vi "Create Bar.vi"(6 "Draw Mode":T1(ring)=enum."Quads", 7 "3D Bar Property":T2, 8 "error in (no error)":errorcluster, 10 "Plot Representation In":T4, 11 "Plot Object In":refnum<vi>) -> (0 "error out":errorcluster, 2 "Plot Representation Out":T4, 3 "Plot Object Out":refnum<vi>, 4 "Sector Object Out":refnum<vi>, 5 "Bar Drawable":refnum<vi>)   [LabVIEW 2017, in "3D Bar.lvclass"]
uses:
  <vilib>/Math Plots/3D Math Plots/3D Bar/3D Bar/3D Bar.lvclass
  <vilib>/Math Plots/3D Math Plots/3D Plot/3D Plot/Typedef/Plot Representation.ctl
  <vilib>/Math Plots/3D Math Plots/3D Plot/3D Plot/Typedef/Range Clusters.ctl
  <vilib>/Math Plots/3D Math Plots/3D Plot/3D Plot/Typedef/Mesh Data.ctl
  <vilib>/Math Plots/3D Math Plots/3D Bar/3D Bar/Typedef/3D Bar Property.ctl
  <vilib>/Math Plots/3D Math Plots/3D Plot/3D Plot/Typedef/Line Type.ctl
  <vilib>/picture/3D Picture Control/Object/Create Object (name).vi
  <vilib>/picture/3D Picture Control/NI_3D Picture Control.lvlib
  <vilib>/Math Plots/3D Math Plots/3D Plot/3D Plot/3D Plot.lvclass
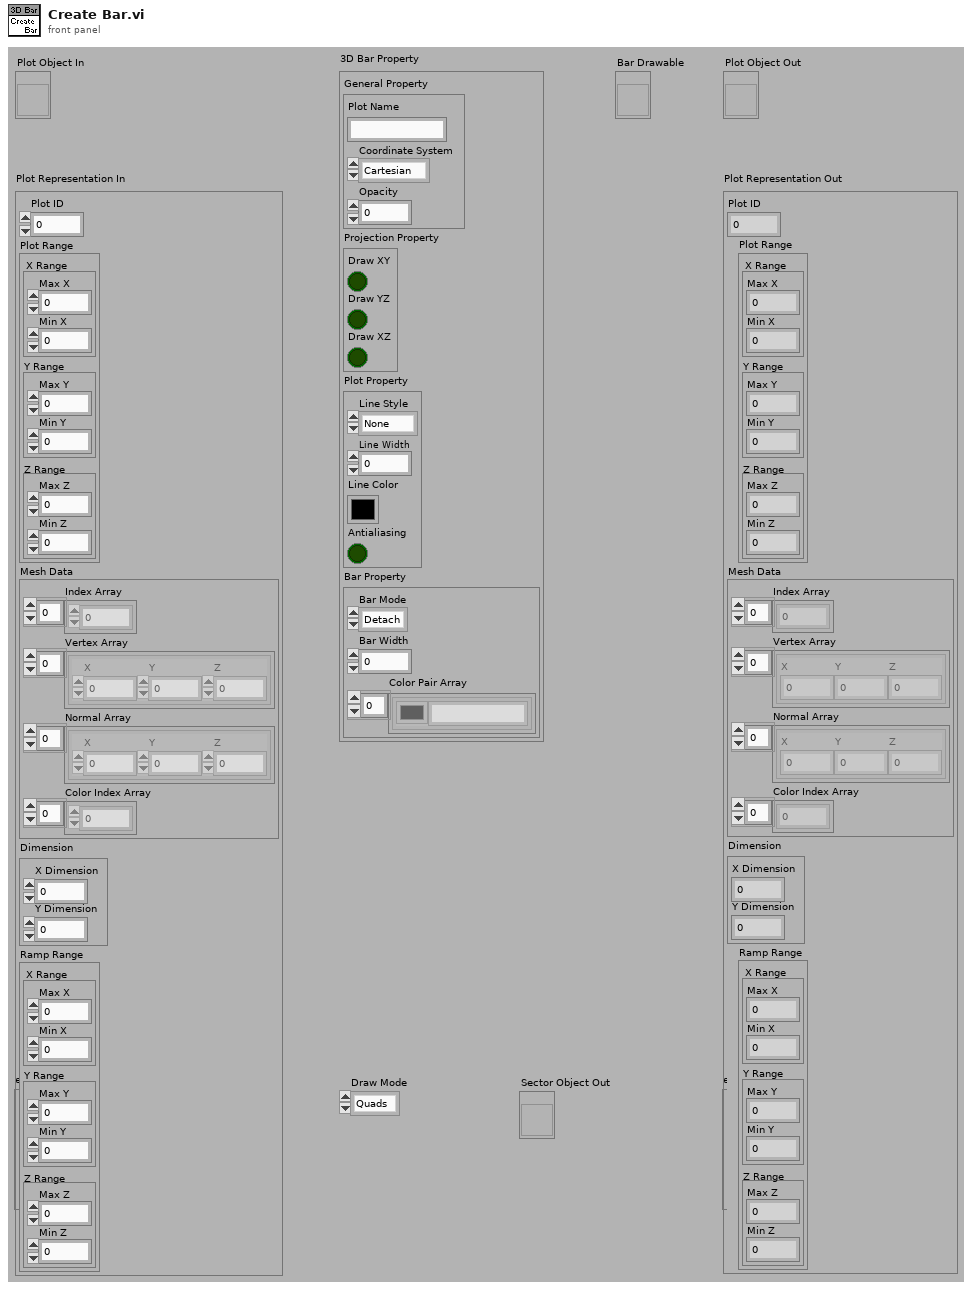
[diagram p1: front panel]
types:
  T1 = enum16{"Points", "Lines", "Line Strip", "Line Loop", "Triangles", "Triangle Strip", "Triangle Fan", "Quads", "Quad Strip", "Polygon"}
  T2 = typedef "3D Bar.lvclass/3D Bar Property.ctl" = cluster{"General Property":cluster{"Plot Name":string, "Coordinate System":enum16{"Cartesian", "Cylindrical", "Spherical"}, "Opacity":sgl}, "Projection Property":cluster{"Draw XY":bool, "Draw YZ":bool, "Draw XZ":bool}, "Plot Property":cluster{"Line Style":T3, "Line Width":sgl, "Line Color":u32, "Antialiasing":bool}, "Bar Property":cluster{"Bar Mode":enum16{"Detach", "Group", "Stack"}, "Bar Width":sgl, "Color Pair Array":cluster{"Color":u32, "String":string}[]}}
  T3 = typedef "3D Plot.lvclass/Line Type.ctl" = enum16{"None", "Solid", "Dash", "Dot", "Dash Dot"}
  T4 = typedef "3D Plot.lvclass/Plot Representation.ctl" = cluster{"Plot ID":i32, "Plot Range":T5, "Mesh Data":T6, "Dimension":cluster{"X Dimension":i32, "Y Dimension":i32}, "Ramp Range":T5}
  T5 = typedef "3D Plot.lvclass/Range Clusters.ctl" = cluster{"X Range":cluster{"Max X":sgl, "Min X":sgl}, "Y Range":cluster{"Max Y":sgl, "Min Y":sgl}, "Z Range":cluster{"Max Z":sgl, "Min Z":sgl}}
  T6 = typedef "3D Plot.lvclass/Mesh Data.ctl" = cluster{"Index Array":u32[], "Vertex Array":cluster{"X":sgl, "Y":sgl, "Z":sgl}[], "Normal Array":cluster{"X":sgl, "Y":sgl, "Z":sgl}[], "Color Index Array":i32[]}
  T7 = enum16{"Inherit Value", "Points", "Wireframe", "Polygons"}
  T8 = enum16{"Inherit Material", "Use entire Material", "Ignore Ambient", "Ignore Diffuse", "Ignore Specular", "Ignore Emission", "Ignore Ambient and Diffuse"}
  T9 = enum16{"Inherit Value", "Counterclockwise", "Clockwise"}
  T10 = enum16{"Overall", "Per Primitive", "Per Vertex", "Binding Off"}
  T11 = enum16{"Normal Bin", "Opaque Bin", "Transparent Bin"}
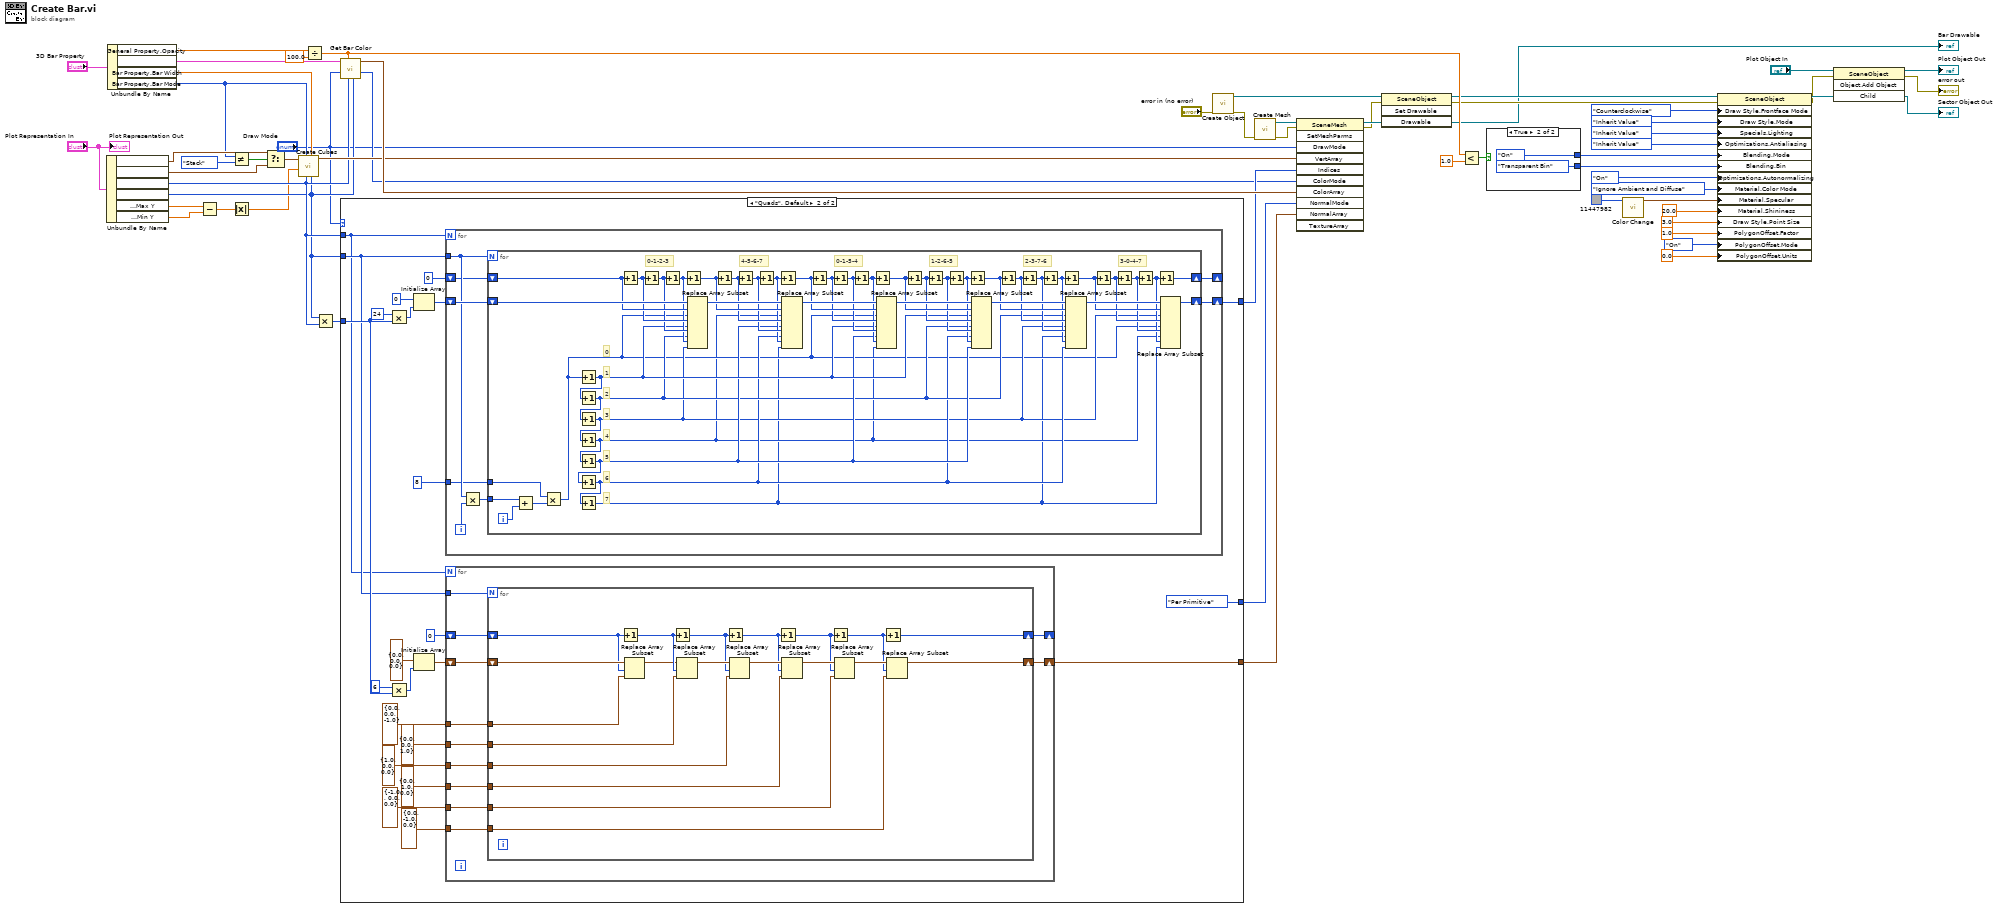
[diagram p0: block diagram]
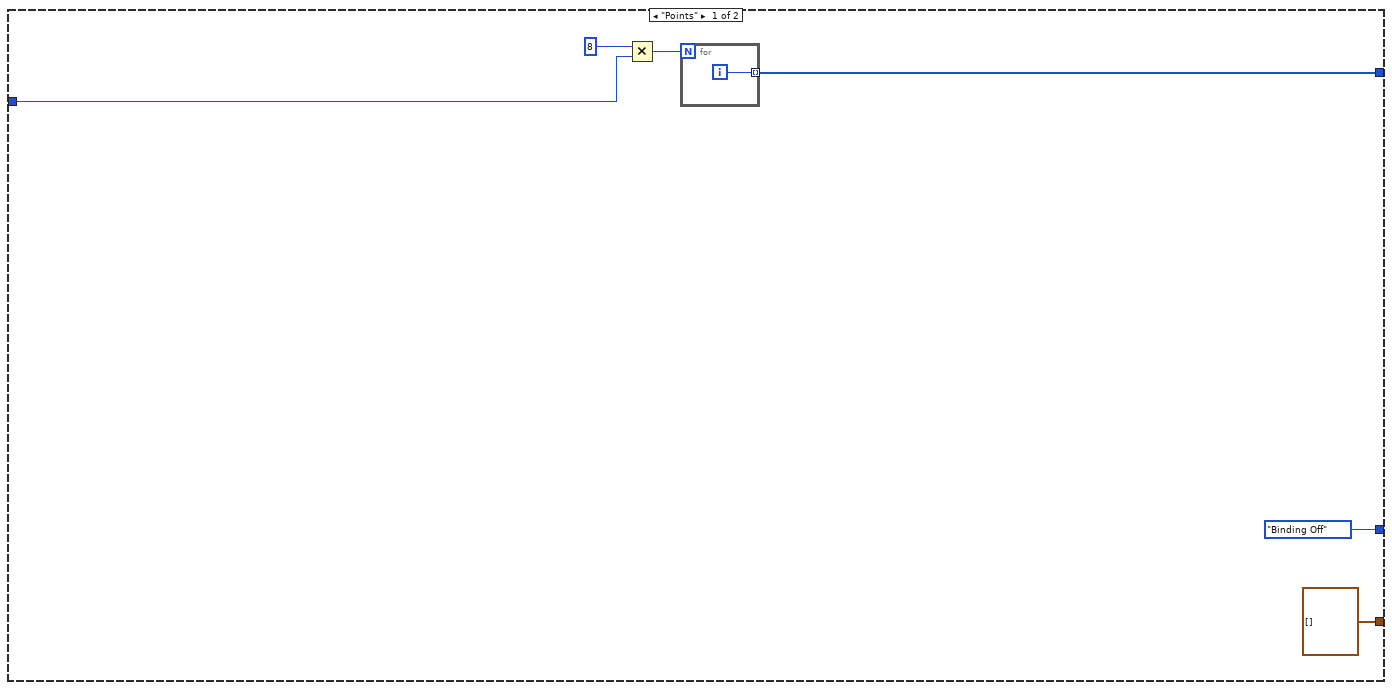
[diagram p2: hidden frame]
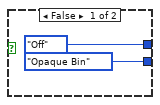
[diagram p3: hidden frame]
diagram:
  n1 = Unbundle By Name("Plot Representation In") -> ("Mesh Data.Vertex Array"=w39:cluster{"X":sgl, "Y":sgl, "Z":sgl}[], "Mesh Data.Normal Array"=w38:cluster{"X":sgl, "Y":sgl, "Z":sgl}[], "Dimension.X Dimension"=w12:i32, "Dimension.Y Dimension"=w11:i32, "Ramp Range.Y Range.Max Y"=w3:sgl, "Ramp Range.Y Range.Min Y"=w2:sgl)
  n2 = Unbundle By Name("3D Bar Property") -> ("General Property.Opacity"=w52:sgl, "Bar Property.Color Pair Array"=w59:cluster{"Color":u32, "String":string}[], "Bar Property.Bar Width"=w54:sgl, "Bar Property.Bar Mode"=w36:enum16{"Detach", "Group", "Stack"})
  n3 = Subtract(x=w3, y=w2) -> (x-y=w4:sgl)
  n4 = Not Equal?(x=w36, y=enum16{"Detach", "Group", "Stack"}."Stack" ("Bar Property.Bar Mode")) -> (x != y?=w40:bool)
  n5 = Absolute Value(x=w4) -> (abs(x)=w1:sgl)
  n6 = Select(t=w39, s=w40, f=w38) -> (s? t:f=w20:cluster{"X":sgl, "Y":sgl, "Z":sgl}[])
  n7 = call <vilib>:"Create Cubes.vi"("Y Dimension"=w11, "Width"=w54, "X Dimension"=w12, "Bar Mode"=w36, "Difference"=w1, "Bar Info In"=w20) -> ("Vertex Array Out"=w19:cluster{"X":sgl, "Y":sgl, "Z":sgl}[])  [unwired: 3 in, 2 out]
  n8 = Divide(x=w52, y=sgl 100.0) -> (x/y=w31:sgl)
  n9 = Multiply(x=w11, y=w12) -> (x*y=w10:i32)
  n10 = call <vilib>:"Get Bar Color.vi"("Y Dimension"=w11, "X Dimension"=w12, "Opacity"=w31, "Draw Mode"="Draw Mode", "Color Pair Array"=w59) -> ("Color Binding Mode"=w9:T10, "Color Array"=w21:cluster{"R":sgl, "G":sgl, "B":sgl, "A":sgl}[])  [unwired: 1 in, 4 out]
  n11 = case shown="\"Quads\", Default" "Draw Mode" {
    tunnel: [w65 w85] -> w13
    tunnel: w12 -> [_ w76]
    tunnel: w11 -> [_ w77]
    tunnel: w10 -> [w66 w79]
    tunnel: [cluster{"X":sgl, "Y":sgl, "Z":sgl}[] [] w69] -> w6
    tunnel: [T10."Binding Off" ("Normal Binding Mode") T10."Per Primitive" ("Normal Binding Mode")] -> w5
    frame "Points" {
      n12 = Multiply(x=8, y=w66) -> (x*y=w64:i32)
      n13 = for {
        N: w64 -> [_]
        tunnel: [w67] -> w65 mode=indexing
        i -> [w67]
      }
    }
    frame "Quads", Default {
      n14 = Multiply(x=24 ("value"), y=w79) -> (x*y=w89:i32)
      n15 = Multiply(x=6 ("value"), y=w79) -> (x*y=w78:i32)
      n16 = Initialize Array(u32 0 ("value"), w89) -> (w88:u32[])
      n17 = Initialize Array(cluster{"X":sgl, "Y":sgl, "Z":sgl} {"X"=0.0, "Y"=0.0, "Z"=0.0} ("3D Point"), w78) -> (w82:cluster{"X":sgl, "Y":sgl, "Z":sgl}[])
      n18 = for {
        N: w76 -> [_]
        shift-right: [w128] -> w85
        shift-left: w88 -> [w129]
        tunnel: w77 -> [w125]
        tunnel: 8 ("value") -> [w124]
        shift-right: [w122] -> _
        shift-left: 0 ("value") -> [w123]
        i -> [w127]
        n19 = Multiply(x=w125, y=w127) -> (x*y=w126:i32)
        n20 = for {
          N: w125 -> [_]
          shift-right: [w163] -> w128
          shift-left: w129 -> [w169]
          tunnel: w126 -> [w173]
          tunnel: w124 -> [w170]
          shift-right: [w162] -> w122
          shift-left: w123 -> [w161]
          i -> [w172]
          # "3-0-4-7"
          # "2-3-7-6"
          # "1-2-6-5"
          # "0-1-5-4"
          # "4-5-6-7"
          # "0-1-2-3"
          # "7"
          # "6"
          # "5"
          # "4"
          # "3"
          # "2"
          # "1"
          # "0"
          n21 = Add(x=w173, y=w172) -> (x+y=w171:i32)
          n22 = Multiply(x=w170, y=w171) -> (x*y=w132:i32)
          n23 = Increment(x=w132) -> (x+1=w137:i32)
          n24 = Increment(x=w137) -> (x+1=w135:i32)
          n25 = Increment(x=w135) -> (x+1=w133:i32)
          n26 = Increment(x=w133) -> (x+1=w131:i32)
          n27 = Increment(x=w131) -> (x+1=w136:i32)
          n28 = Increment(x=w136) -> (x+1=w134:i32)
          n29 = Increment(x=w134) -> (x+1=w130:i32)
          n30 = Increment(x=w161) -> (x+1=w160:i32)
          n31 = Increment(x=w160) -> (x+1=w159:i32)
          n32 = Increment(x=w159) -> (x+1=w158:i32)
          n33 = Increment(x=w158) -> (x+1=w157:i32)
          n34 = Replace Array Subset(array=w169, new element #1=w132, index #1=w161, new element #2=w137, index #2=w160, new element #3=w135, index #3=w159, new element #4=w133, index #4=w158) -> (w168:u32[])
          n35 = Increment(x=w157) -> (x+1=w156:i32)
          n36 = Increment(x=w156) -> (x+1=w155:i32)
          n37 = Increment(x=w155) -> (x+1=w154:i32)
          n38 = Increment(x=w154) -> (x+1=w153:i32)
          n39 = Replace Array Subset(array=w168, new element #1=w131, index #1=w157, new element #2=w136, index #2=w156, new element #3=w134, index #3=w155, new element #4=w130, index #4=w154) -> (w167:u32[])
          n40 = Increment(x=w153) -> (x+1=w152:i32)
          n41 = Increment(x=w152) -> (x+1=w151:i32)
          n42 = Increment(x=w151) -> (x+1=w150:i32)
          n43 = Increment(x=w150) -> (x+1=w149:i32)
          n44 = Replace Array Subset(array=w167, new element #1=w132, index #1=w153, new element #2=w137, index #2=w152, new element #3=w136, index #3=w151, new element #4=w131, index #4=w150) -> (w166:u32[])
          n45 = Increment(x=w149) -> (x+1=w148:i32)
          n46 = Increment(x=w148) -> (x+1=w147:i32)
          n47 = Increment(x=w147) -> (x+1=w146:i32)
          n48 = Increment(x=w146) -> (x+1=w145:i32)
          n49 = Replace Array Subset(array=w166, new element #1=w137, index #1=w149, new element #2=w135, index #2=w148, new element #3=w134, index #3=w147, new element #4=w136, index #4=w146) -> (w165:u32[])
          n50 = Increment(x=w145) -> (x+1=w144:i32)
          n51 = Increment(x=w144) -> (x+1=w143:i32)
          n52 = Increment(x=w143) -> (x+1=w142:i32)
          n53 = Increment(x=w142) -> (x+1=w141:i32)
          n54 = Replace Array Subset(array=w165, new element #1=w135, index #1=w145, new element #2=w133, index #2=w144, new element #3=w130, index #3=w143, new element #4=w134, index #4=w142) -> (w164:u32[])
          n55 = Increment(x=w141) -> (x+1=w140:i32)
          n56 = Increment(x=w140) -> (x+1=w139:i32)
          n57 = Increment(x=w139) -> (x+1=w138:i32)
          n58 = Increment(x=w138) -> (x+1=w162:i32)
          n59 = Replace Array Subset(array=w164, new element #1=w133, index #1=w141, new element #2=w132, index #2=w140, new element #3=w131, index #3=w139, new element #4=w130, index #4=w138) -> (w163:u32[])
        }
      }
      n60 = for {
        N: w76 -> [_]
        tunnel: w77 -> [w101]
        shift-right: [w98] -> w69
        shift-left: w82 -> [w100]
        shift-right: [w97] -> _
        shift-left: 0 -> [w99]
        tunnel: cluster{"X":sgl, "Y":sgl, "Z":sgl} {"X"=0.0, "Y"=0.0, "Z"=-1.0} ("3D Point") -> [w96]
        tunnel: cluster{"X":sgl, "Y":sgl, "Z":sgl} {"X"=0.0, "Y"=0.0, "Z"=1.0} ("3D Point") -> [w95]
        tunnel: cluster{"X":sgl, "Y":sgl, "Z":sgl} {"X"=1.0, "Y"=0.0, "Z"=0.0} ("3D Point") -> [w94]
        tunnel: cluster{"X":sgl, "Y":sgl, "Z":sgl} {"X"=0.0, "Y"=1.0, "Z"=0.0} ("3D Point") -> [w93]
        tunnel: cluster{"X":sgl, "Y":sgl, "Z":sgl} {"X"=0.0, "Y"=-1.0, "Z"=0.0} ("3D Point") -> [w91]
        tunnel: cluster{"X":sgl, "Y":sgl, "Z":sgl} {"X"=-1.0, "Y"=0.0, "Z"=0.0} ("3D Point") -> [w92]
        n61 = for {
          N: w101 -> [_]
          shift-right: [w112] -> w98
          shift-left: w100 -> [w121]
          shift-right: [w120] -> w97
          shift-left: w99 -> [w119]
          tunnel: w96 -> [w107]
          tunnel: w95 -> [w106]
          tunnel: w94 -> [w105]
          tunnel: w93 -> [w104]
          tunnel: w92 -> [w103]
          tunnel: w91 -> [w102]
          n62 = Increment(x=w119) -> (x+1=w118:i32)
          n63 = Replace Array Subset(array=w121, new element=w107, index=w119) -> (w117:cluster{"X":sgl, "Y":sgl, "Z":sgl}[])
          n64 = Increment(x=w118) -> (x+1=w111:i32)
          n65 = Replace Array Subset(array=w117, new element=w106, index=w118) -> (w116:cluster{"X":sgl, "Y":sgl, "Z":sgl}[])
          n66 = Increment(x=w111) -> (x+1=w110:i32)
          n67 = Replace Array Subset(array=w116, new element=w105, index=w111) -> (w115:cluster{"X":sgl, "Y":sgl, "Z":sgl}[])
          n68 = Increment(x=w110) -> (x+1=w109:i32)
          n69 = Replace Array Subset(array=w115, new element=w104, index=w110) -> (w114:cluster{"X":sgl, "Y":sgl, "Z":sgl}[])
          n70 = Increment(x=w109) -> (x+1=w108:i32)
          n71 = Replace Array Subset(array=w114, new element=w103, index=w109) -> (w113:cluster{"X":sgl, "Y":sgl, "Z":sgl}[])
          n72 = Increment(x=w108) -> (x+1=w120:i32)
          n73 = Replace Array Subset(array=w113, new element=w102, index=w108) -> (w112:cluster{"X":sgl, "Y":sgl, "Z":sgl}[])
        }
      }
    }
  }
  n74 = call-poly <vilib>:"Create Object.vi"("error in (no error)"="error in (no error)") -> ("error out"=w15:errorcluster, "Scene:New Object"=w18:refnum<vi>)  [unwired: 9 in]
  n75 = call <vilib>:"Create Mesh.vi"("error in (no error)"=w15) -> ("error out"=w22:errorcluster, "New Mesh Refnum"=w25:refnum<vi>)  [unwired: 9 in]
  n76 = invoke class="SceneMesh" method="SetMeshParms"(reference=w25, error in=w22, "DrawMode"="Draw Mode", "VertArray"=w19, "Indices"=w13, "ColorMode"=w9, "ColorArray"=w21, "NormalMode"=w5, "NormalArray"=w6) -> (reference out=w24:refnum<vi>, error out=w23:errorcluster)  [unwired: 2 in, 9 out]
  n77 = invoke class="SceneObject" method="Set Drawable"(reference=w18, error in=w23, "Drawable"=w24) -> (reference out=w17:refnum<vi>, error out=w14:errorcluster, "Drawable"=→"Bar Drawable":refnum<vi>)  [unwired: 1 in, 1 out]
  n78 = Less?(x=w31, y=sgl 1.0) -> (x < y?=w34:bool)
  n79 = case shown="True" w34 {
    tunnel: [T11."Opaque Bin" ("Blending:Bin") T11."Transparent Bin" ("Blending:Bin")] -> w32
    tunnel: [enum16{"Inherit Value", "Off", "On"}."Off" ("Blending:Mode") enum16{"Inherit Value", "Off", "On"}."On" ("Blending:Mode")] -> w33
    frame False {
    }
    frame True {
    }
  }
  n80 = call <vilib>:"Color Change.vi"("Color"=u32 11447982) -> ("RGBA"=w48:cluster{"R":sgl, "G":sgl, "B":sgl, "A":sgl})  [unwired: 1 in, 9 out]
  n81 = property class="SceneObject"(reference=w17, error in=w14, "Draw Style.Frontface Mode"=T9."Counterclockwise" ("Draw Style:Frontface Mode"), "Draw Style.Mode"=T7."Inherit Value" ("Draw Style:Mode"), "Specials.Lighting"=enum16{"Inherit Value", "Off", "On"}."Inherit Value" ("Specials:Lighting"), "Optimizations.Antialiasing"=enum16{"Inherit Value", "Off", "On"}."Inherit Value" ("Optimizations:Antialiasing"), "Blending.Mode"=w33, "Blending.Bin"=w32, "Optimizations.Autonormalizing"=enum16{"Inherit Value", "Off", "On"}."On" ("Optimizations:Autonormalizing"), "Material.Color Mode"=T8."Ignore Ambient and Diffuse" ("Material:Color Mode"), "Material.Specular"=w48, "Material.Shininess"=sgl 20.0 ("Material:Shininess"), "Draw Style.Point Size"=sgl 3.0 ("Draw Style:Point Size"), "PolygonOffset.Factor"=sgl 1.0 ("PolygonOffset:Factor"), "PolygonOffset.Mode"=enum16{"Inherit Value", "Off", "On"}."On" ("PolygonOffset:Mode"), "PolygonOffset.Units"=sgl 0.0 ("PolygonOffset:Units")) -> (reference out=w41:refnum<vi>, error out=w26:errorcluster)
  n82 = invoke class="SceneObject" method="Object.Add Object"(reference="Plot Object In", error in=w26, "Child"=w41) -> (reference out=→"Plot Object Out":refnum<vi>, error out=→"error out":errorcluster, "Child"=→"Sector Object Out":refnum<vi>)  [unwired: 1 in, 1 out]
  "Plot Representation Out" <- "Plot Representation In"
